vi "Append (SubVI).vi"(8 "error in (no error)":errorcluster, 10 "read buffer":string, 11 "file (use dialog)":path) -> (0 "error out":errorcluster)   [LabVIEW 2019]
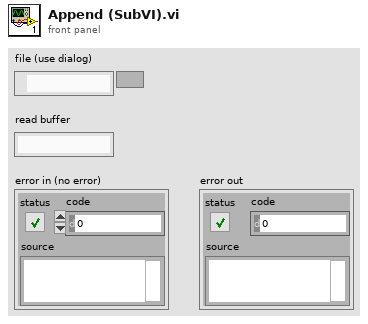
[diagram p1: front panel]
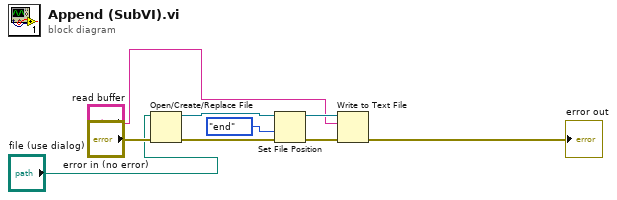
[diagram p0: block diagram]
diagram:
  n1 = Open/Create/Replace File(file path (use dialog)="file (use dialog)", error in="error in (no error)") -> (refnum out=w4:refnum<file>, error out=w3:errorcluster)  [unwired: 4 in, 1 out]
  n2 = Set File Position(refnum=w4, from (0:start)=enum16{"start", "end", "current"}."end", error in=w3) -> (refnum out=w9:refnum<file>, error out=w7:errorcluster)  [unwired: 1 in]
  n3 = Write to Text File(file (use dialog)=w9, text="read buffer", error in=w7) -> (error out=→"error out":errorcluster)  [unwired: 1 in, 2 out]
